vi "Step2to3.vi"   [LabVIEW 2019]
uses:
  Global Var.vi
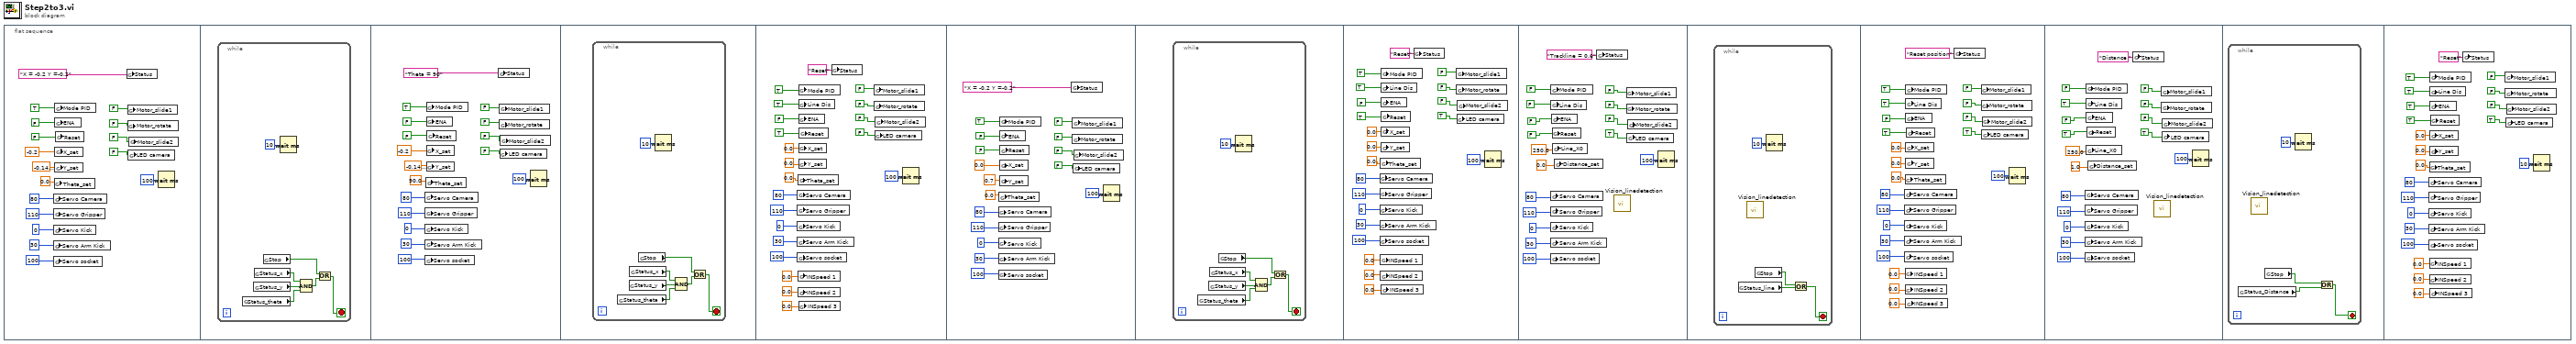
[diagram p0: block diagram]
diagram:
  n1 = flat-sequence {
    frame #0 {
      n2 = global write "Global Var.vi" "Servo Camera"(u8 80 ("Servo Camera")) -> ()
      n3 = global write "Global Var.vi" "Servo Gripper"(u8 110 ("Servo Camera")) -> ()
      n4 = global write "Global Var.vi" "Servo Kick"(u8 0 ("Servo Camera")) -> ()
      n5 = global write "Global Var.vi" "Servo Arm Kick"(u8 30 ("Servo Camera")) -> ()
      n6 = global write "Global Var.vi" "Servo socket"(u8 100 ("Servo Camera")) -> ()
      n7 = global write "Global Var.vi" "Theta_set"(0.0 ("Theta_set")) -> ()
      n8 = global write "Global Var.vi" "Mode PID"(TRUE ("Mode PID")) -> ()
      n9 = global write "Global Var.vi" "ENA"(FALSE ("ENA")) -> ()
      n10 = global write "Global Var.vi" "X_set"(-0.2 ("X_set")) -> ()
      n11 = global write "Global Var.vi" "Y_set"(-0.14999999999999997 ("Y_set")) -> ()
      n12 = global write "Global Var.vi" "Reset"(FALSE ("ENA")) -> ()
      n13 = global write "Global Var.vi" "Status"("X = -0.2 Y =-0.2" ("Status")) -> ()
      n14 = global write "Global Var.vi" "Motor_slide1"(FALSE ("Mode PID")) -> ()
      n15 = global write "Global Var.vi" "Motor_rotate"(FALSE ("ENA")) -> ()
      n16 = global write "Global Var.vi" "LED camera"(FALSE ("LED camera")) -> ()
      n17 = global write "Global Var.vi" "Motor_slide2"(FALSE ("ENA")) -> ()
      n18 = Wait (ms)(milliseconds to wait=u32 100) -> ()  [unwired: 1 out]
    }
    frame #1 {
      n19 = while {
        stop <- w20 stop-if-true
        n20 = global read "Global Var.vi" "Status_theta"() -> (w22:bool)
        n21 = global read "Global Var.vi" "Status_y"() -> (w24:bool)
        n22 = global read "Global Var.vi" "Status_x"() -> (w23:bool)
        n23 = global read "Global Var.vi" "Stop"() -> (w18:bool)
        n24 = Wait (ms)(milliseconds to wait=u32 10) -> ()  [unwired: 1 out]
        n25 = Compound Arithmetic op=AND(w23, w24, w22) -> (w19:bool)
        n26 = Or(x=w18, y=w19) -> (x .or. y?=w20:bool)
      }
    }
    frame #2 {
      n27 = global write "Global Var.vi" "Servo Camera"(u8 80 ("Servo Camera")) -> ()
      n28 = global write "Global Var.vi" "Servo Gripper"(u8 110 ("Servo Camera")) -> ()
      n29 = global write "Global Var.vi" "Servo Kick"(u8 0 ("Servo Camera")) -> ()
      n30 = global write "Global Var.vi" "Servo Arm Kick"(u8 30 ("Servo Camera")) -> ()
      n31 = global write "Global Var.vi" "Servo socket"(u8 100 ("Servo Camera")) -> ()
      n32 = global write "Global Var.vi" "Theta_set"(90.0 ("Theta_set")) -> ()
      n33 = global write "Global Var.vi" "Mode PID"(TRUE ("Mode PID")) -> ()
      n34 = global write "Global Var.vi" "ENA"(FALSE ("ENA")) -> ()
      n35 = global write "Global Var.vi" "X_set"(-0.2 ("X_set")) -> ()
      n36 = global write "Global Var.vi" "Y_set"(-0.14999999999999997 ("Y_set")) -> ()
      n37 = global write "Global Var.vi" "Reset"(FALSE ("ENA")) -> ()
      n38 = global write "Global Var.vi" "Status"("Theta = 90" ("Status")) -> ()
      n39 = global write "Global Var.vi" "Motor_slide1"(FALSE ("Mode PID")) -> ()
      n40 = global write "Global Var.vi" "Motor_rotate"(FALSE ("ENA")) -> ()
      n41 = global write "Global Var.vi" "LED camera"(FALSE ("LED camera")) -> ()
      n42 = global write "Global Var.vi" "Motor_slide2"(FALSE ("ENA")) -> ()
      n43 = Wait (ms)(milliseconds to wait=u32 100) -> ()  [unwired: 1 out]
    }
    frame #3 {
      n44 = while {
        stop <- w44 stop-if-true
        n45 = global read "Global Var.vi" "Status_theta"() -> (w46:bool)
        n46 = global read "Global Var.vi" "Status_y"() -> (w48:bool)
        n47 = global read "Global Var.vi" "Status_x"() -> (w47:bool)
        n48 = global read "Global Var.vi" "Stop"() -> (w42:bool)
        n49 = Wait (ms)(milliseconds to wait=u32 10) -> ()  [unwired: 1 out]
        n50 = Compound Arithmetic op=AND(w47, w48, w46) -> (w43:bool)
        n51 = Or(x=w42, y=w43) -> (x .or. y?=w44:bool)
      }
    }
    frame #4 {
      n52 = global write "Global Var.vi" "Servo Camera"(u8 80 ("Servo Camera")) -> ()
      n53 = global write "Global Var.vi" "Servo Gripper"(u8 110 ("Servo Camera")) -> ()
      n54 = global write "Global Var.vi" "Servo Kick"(u8 0 ("Servo Camera")) -> ()
      n55 = global write "Global Var.vi" "Servo Arm Kick"(u8 30 ("Servo Camera")) -> ()
      n56 = global write "Global Var.vi" "Servo socket"(u8 100 ("Servo Camera")) -> ()
      n57 = global write "Global Var.vi" "Theta_set"(0.0 ("Theta_set")) -> ()
      n58 = global write "Global Var.vi" "INSpeed 1"(0.0 ("X_set")) -> ()
      n59 = global write "Global Var.vi" "INSpeed 2"(0.0 ("Y_set")) -> ()
      n60 = global write "Global Var.vi" "Mode PID"(TRUE ("Mode PID")) -> ()
      n61 = global write "Global Var.vi" "Line Dis"(TRUE ("Mode PID")) -> ()
      n62 = global write "Global Var.vi" "ENA"(FALSE ("ENA")) -> ()
      n63 = global write "Global Var.vi" "X_set"(0.0 ("X_set")) -> ()
      n64 = global write "Global Var.vi" "Y_set"(0.0 ("Y_set")) -> ()
      n65 = global write "Global Var.vi" "INSpeed 3"(0.0 ("Theta_set")) -> ()
      n66 = global write "Global Var.vi" "Reset"(TRUE ("ENA")) -> ()
      n67 = global write "Global Var.vi" "Status"("Reset" ("Status")) -> ()
      n68 = global write "Global Var.vi" "Motor_slide1"(FALSE ("Mode PID")) -> ()
      n69 = global write "Global Var.vi" "Motor_rotate"(FALSE ("ENA")) -> ()
      n70 = global write "Global Var.vi" "LED camera"(FALSE ("LED camera")) -> ()
      n71 = global write "Global Var.vi" "Motor_slide2"(FALSE ("ENA")) -> ()
      n72 = Wait (ms)(milliseconds to wait=u32 100) -> ()  [unwired: 1 out]
    }
    frame #5 {
      n73 = global write "Global Var.vi" "Servo Camera"(u8 80 ("Servo Camera")) -> ()
      n74 = global write "Global Var.vi" "Servo Gripper"(u8 110 ("Servo Camera")) -> ()
      n75 = global write "Global Var.vi" "Servo Kick"(u8 0 ("Servo Camera")) -> ()
      n76 = global write "Global Var.vi" "Servo Arm Kick"(u8 30 ("Servo Camera")) -> ()
      n77 = global write "Global Var.vi" "Servo socket"(u8 100 ("Servo Camera")) -> ()
      n78 = global write "Global Var.vi" "Theta_set"(0.0 ("Theta_set")) -> ()
      n79 = global write "Global Var.vi" "Mode PID"(TRUE ("Mode PID")) -> ()
      n80 = global write "Global Var.vi" "ENA"(FALSE ("ENA")) -> ()
      n81 = global write "Global Var.vi" "X_set"(0.0 ("X_set")) -> ()
      n82 = global write "Global Var.vi" "Y_set"(0.7 ("Y_set")) -> ()
      n83 = global write "Global Var.vi" "Reset"(FALSE ("ENA")) -> ()
      n84 = global write "Global Var.vi" "Status"("X = -0.2 Y =-0.2" ("Status")) -> ()
      n85 = global write "Global Var.vi" "Motor_slide1"(FALSE ("Mode PID")) -> ()
      n86 = global write "Global Var.vi" "Motor_rotate"(FALSE ("ENA")) -> ()
      n87 = global write "Global Var.vi" "LED camera"(FALSE ("LED camera")) -> ()
      n88 = global write "Global Var.vi" "Motor_slide2"(FALSE ("ENA")) -> ()
      n89 = Wait (ms)(milliseconds to wait=u32 100) -> ()  [unwired: 1 out]
    }
    frame #6 {
      n90 = while {
        stop <- w89 stop-if-true
        n91 = global read "Global Var.vi" "Status_theta"() -> (w91:bool)
        n92 = global read "Global Var.vi" "Status_y"() -> (w93:bool)
        n93 = global read "Global Var.vi" "Status_x"() -> (w92:bool)
        n94 = global read "Global Var.vi" "Stop"() -> (w87:bool)
        n95 = Wait (ms)(milliseconds to wait=u32 10) -> ()  [unwired: 1 out]
        n96 = Compound Arithmetic op=AND(w92, w93, w91) -> (w88:bool)
        n97 = Or(x=w87, y=w88) -> (x .or. y?=w89:bool)
      }
    }
    frame #7 {
      n98 = global write "Global Var.vi" "Servo Camera"(u8 80 ("Servo Camera")) -> ()
      n99 = global write "Global Var.vi" "Servo Gripper"(u8 110 ("Servo Camera")) -> ()
      n100 = global write "Global Var.vi" "Servo Kick"(u8 0 ("Servo Camera")) -> ()
      n101 = global write "Global Var.vi" "Servo Arm Kick"(u8 30 ("Servo Camera")) -> ()
      n102 = global write "Global Var.vi" "Servo socket"(u8 100 ("Servo Camera")) -> ()
      n103 = global write "Global Var.vi" "Theta_set"(0.0 ("Theta_set")) -> ()
      n104 = global write "Global Var.vi" "INSpeed 1"(0.0 ("X_set")) -> ()
      n105 = global write "Global Var.vi" "INSpeed 2"(0.0 ("Y_set")) -> ()
      n106 = global write "Global Var.vi" "Mode PID"(TRUE ("Mode PID")) -> ()
      n107 = global write "Global Var.vi" "Line Dis"(TRUE ("Mode PID")) -> ()
      n108 = global write "Global Var.vi" "ENA"(FALSE ("ENA")) -> ()
      n109 = global write "Global Var.vi" "X_set"(0.0 ("X_set")) -> ()
      n110 = global write "Global Var.vi" "Y_set"(0.0 ("Y_set")) -> ()
      n111 = global write "Global Var.vi" "INSpeed 3"(0.0 ("Theta_set")) -> ()
      n112 = global write "Global Var.vi" "Reset"(TRUE ("ENA")) -> ()
      n113 = global write "Global Var.vi" "Status"("Reset" ("Status")) -> ()
      n114 = global write "Global Var.vi" "Motor_slide1"(FALSE ("Mode PID")) -> ()
      n115 = global write "Global Var.vi" "Motor_rotate"(FALSE ("ENA")) -> ()
      n116 = global write "Global Var.vi" "LED camera"(TRUE ("LED camera")) -> ()
      n117 = global write "Global Var.vi" "Motor_slide2"(FALSE ("ENA")) -> ()
      n118 = Wait (ms)(milliseconds to wait=u32 100) -> ()  [unwired: 1 out]
    }
    frame #8 {
      n119 = global write "Global Var.vi" "Servo Camera"(u8 80 ("Servo Camera")) -> ()
      n120 = global write "Global Var.vi" "Servo Gripper"(u8 110 ("Servo Camera")) -> ()
      n121 = global write "Global Var.vi" "Servo Kick"(u8 0 ("Servo Camera")) -> ()
      n122 = global write "Global Var.vi" "Servo Arm Kick"(u8 30 ("Servo Camera")) -> ()
      n123 = global write "Global Var.vi" "Servo socket"(u8 100 ("Servo Camera")) -> ()
      n124 = global write "Global Var.vi" "Mode PID"(FALSE ("Mode PID")) -> ()
      n125 = global write "Global Var.vi" "Line Dis"(FALSE ("Mode PID")) -> ()
      n126 = global write "Global Var.vi" "ENA"(FALSE ("ENA")) -> ()
      n127 = global write "Global Var.vi" "Reset"(FALSE ("ENA")) -> ()
      n128 = global write "Global Var.vi" "Line_X0"(250.0 ("Y_set")) -> ()
      n129 = global write "Global Var.vi" "Distance_set"(0.0 ("Y_set")) -> ()
      n130 = global write "Global Var.vi" "Status"("Trackline = 0.6" ("Status")) -> ()
      n131 = call "Vision_linedetection.vi"() -> ()  [unwired: 12 in]
      n132 = global write "Global Var.vi" "Motor_slide1"(FALSE ("Mode PID")) -> ()
      n133 = global write "Global Var.vi" "Motor_rotate"(FALSE ("ENA")) -> ()
      n134 = global write "Global Var.vi" "LED camera"(TRUE ("LED camera")) -> ()
      n135 = global write "Global Var.vi" "Motor_slide2"(FALSE ("ENA")) -> ()
      n136 = Wait (ms)(milliseconds to wait=u32 100) -> ()  [unwired: 1 out]
    }
    frame #9 {
      n137 = while {
        stop <- w133 stop-if-true
        n138 = global read "Global Var.vi" "Status_line"() -> (w134:bool)
        n139 = call "Vision_linedetection.vi"() -> ()  [unwired: 12 in]
        n140 = global read "Global Var.vi" "Stop"() -> (w132:bool)
        n141 = Wait (ms)(milliseconds to wait=u32 10) -> ()  [unwired: 1 out]
        n142 = Or(x=w132, y=w134) -> (x .or. y?=w133:bool)
      }
    }
    frame #10 {
      n143 = global write "Global Var.vi" "Servo Camera"(u8 80 ("Servo Camera")) -> ()
      n144 = global write "Global Var.vi" "Servo Gripper"(u8 110 ("Servo Camera")) -> ()
      n145 = global write "Global Var.vi" "Servo Kick"(u8 0 ("Servo Camera")) -> ()
      n146 = global write "Global Var.vi" "Servo Arm Kick"(u8 30 ("Servo Camera")) -> ()
      n147 = global write "Global Var.vi" "Servo socket"(u8 100 ("Servo Camera")) -> ()
      n148 = global write "Global Var.vi" "Theta_set"(0.0 ("Theta_set")) -> ()
      n149 = global write "Global Var.vi" "INSpeed 1"(0.0 ("X_set")) -> ()
      n150 = global write "Global Var.vi" "INSpeed 2"(0.0 ("Y_set")) -> ()
      n151 = global write "Global Var.vi" "Mode PID"(TRUE ("Mode PID")) -> ()
      n152 = global write "Global Var.vi" "Line Dis"(TRUE ("Mode PID")) -> ()
      n153 = global write "Global Var.vi" "ENA"(FALSE ("ENA")) -> ()
      n154 = global write "Global Var.vi" "X_set"(0.0 ("X_set")) -> ()
      n155 = global write "Global Var.vi" "Y_set"(0.0 ("Y_set")) -> ()
      n156 = global write "Global Var.vi" "INSpeed 3"(0.0 ("Theta_set")) -> ()
      n157 = global write "Global Var.vi" "Reset"(TRUE ("ENA")) -> ()
      n158 = global write "Global Var.vi" "Status"("Reset position" ("Status")) -> ()
      n159 = global write "Global Var.vi" "Motor_slide1"(FALSE ("Mode PID")) -> ()
      n160 = global write "Global Var.vi" "Motor_rotate"(FALSE ("ENA")) -> ()
      n161 = global write "Global Var.vi" "LED camera"(TRUE ("LED camera")) -> ()
      n162 = global write "Global Var.vi" "Motor_slide2"(FALSE ("ENA")) -> ()
      n163 = Wait (ms)(milliseconds to wait=u32 100) -> ()  [unwired: 1 out]
    }
    frame #11 {
      n164 = global write "Global Var.vi" "Servo Camera"(u8 80 ("Servo Camera")) -> ()
      n165 = global write "Global Var.vi" "Servo Gripper"(u8 110 ("Servo Camera")) -> ()
      n166 = global write "Global Var.vi" "Servo Kick"(u8 0 ("Servo Camera")) -> ()
      n167 = global write "Global Var.vi" "Servo Arm Kick"(u8 30 ("Servo Camera")) -> ()
      n168 = global write "Global Var.vi" "Servo socket"(u8 100 ("Servo Camera")) -> ()
      n169 = global write "Global Var.vi" "Mode PID"(FALSE ("Mode PID")) -> ()
      n170 = global write "Global Var.vi" "Line Dis"(TRUE ("Mode PID")) -> ()
      n171 = global write "Global Var.vi" "ENA"(FALSE ("ENA")) -> ()
      n172 = global write "Global Var.vi" "Line_X0"(250.0 ("Y_set")) -> ()
      n173 = global write "Global Var.vi" "Reset"(TRUE ("ENA")) -> ()
      n174 = global write "Global Var.vi" "Distance_set"(1.0 ("Y_set")) -> ()
      n175 = global write "Global Var.vi" "Status"("Distance " ("Status")) -> ()
      n176 = call "Vision_linedetection.vi"() -> ()  [unwired: 12 in]
      n177 = global write "Global Var.vi" "Motor_slide1"(FALSE ("Mode PID")) -> ()
      n178 = global write "Global Var.vi" "Motor_rotate"(FALSE ("ENA")) -> ()
      n179 = global write "Global Var.vi" "LED camera"(TRUE ("LED camera")) -> ()
      n180 = global write "Global Var.vi" "Motor_slide2"(FALSE ("ENA")) -> ()
      n181 = Wait (ms)(milliseconds to wait=u32 100) -> ()  [unwired: 1 out]
    }
    frame #12 {
      n182 = while {
        stop <- w176 stop-if-true
        n183 = global read "Global Var.vi" "Status_Distance"() -> (w174:bool)
        n184 = call "Vision_linedetection.vi"() -> ()  [unwired: 12 in]
        n185 = global read "Global Var.vi" "Stop"() -> (w175:bool)
        n186 = Wait (ms)(milliseconds to wait=u32 10) -> ()  [unwired: 1 out]
        n187 = Or(x=w175, y=w174) -> (x .or. y?=w176:bool)
      }
    }
    frame #13 {
      n188 = global write "Global Var.vi" "Servo Camera"(u8 80 ("Servo Camera")) -> ()
      n189 = global write "Global Var.vi" "Servo Gripper"(u8 110 ("Servo Camera")) -> ()
      n190 = global write "Global Var.vi" "Servo Kick"(u8 0 ("Servo Camera")) -> ()
      n191 = global write "Global Var.vi" "Servo Arm Kick"(u8 30 ("Servo Camera")) -> ()
      n192 = global write "Global Var.vi" "Servo socket"(u8 100 ("Servo Camera")) -> ()
      n193 = global write "Global Var.vi" "Theta_set"(0.0 ("Theta_set")) -> ()
      n194 = global write "Global Var.vi" "INSpeed 1"(0.0 ("X_set")) -> ()
      n195 = global write "Global Var.vi" "INSpeed 2"(0.0 ("Y_set")) -> ()
      n196 = global write "Global Var.vi" "Mode PID"(TRUE ("Mode PID")) -> ()
      n197 = global write "Global Var.vi" "Line Dis"(TRUE ("Mode PID")) -> ()
      n198 = global write "Global Var.vi" "ENA"(TRUE ("ENA")) -> ()
      n199 = global write "Global Var.vi" "X_set"(0.0 ("X_set")) -> ()
      n200 = global write "Global Var.vi" "Y_set"(0.0 ("Y_set")) -> ()
      n201 = global write "Global Var.vi" "INSpeed 3"(0.0 ("Theta_set")) -> ()
      n202 = global write "Global Var.vi" "Reset"(TRUE ("ENA")) -> ()
      n203 = global write "Global Var.vi" "Status"("Reset" ("Status")) -> ()
      n204 = global write "Global Var.vi" "Motor_slide1"(FALSE ("Mode PID")) -> ()
      n205 = global write "Global Var.vi" "Motor_rotate"(FALSE ("ENA")) -> ()
      n206 = global write "Global Var.vi" "LED camera"(TRUE ("LED camera")) -> ()
      n207 = global write "Global Var.vi" "Motor_slide2"(FALSE ("ENA")) -> ()
      n208 = Wait (ms)(milliseconds to wait=u32 10) -> ()  [unwired: 1 out]
    }
  }
